vi "3DS Models.vi"(11 "Model":T1=enum."Utah Teapot") -> (3 "Model Out":T2 {"NormalList"."z" format="%.2f"; "NormalList"."y" format="%.2f"; "NormalList"."x" format="%.2f"; "VertexList"."z" format="%.2f"; "VertexList"."y" format="%.2f"; "VertexList"."x" format="%.2f"})   [LabVIEW 2026, in "XRay Part Sample.lvclass"]
uses:
  XRay Part Sample.lvclass
  <vilib>/picture/3D Picture Control/Old 3D Toolkit.llb/model.ctl
  <vilib>/picture/3D Picture Control/Old 3D Toolkit.llb/point3f.ctl
  <vilib>/picture/3D Picture Control/Old 3D Toolkit.llb/VertexMode.ctl
  3D utilities/3DS Models.ctl
  <vilib>/picture/3D Picture Control/NI_Old 3D Toolkit.lvlib
  3D utilities/3D utilities.lvlib
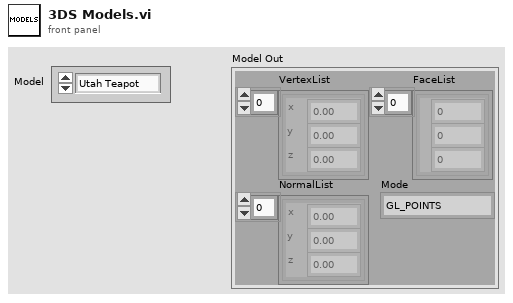
[diagram p1: front panel]
types:
  T1 = typedef "3DS Models.ctl" = enum16{"ASTM E2597 Step Wedge", "NI Bottle", "Utah Teapot", "Utah Teapot (Low Res)", "My Cube", "Tree", "Tree 2", "FreeCAD Sample", "Schenkel", "Bunny", "Corona Virus", "Corona Virus (Low Res)", "Offset"}
  T2 = typedef "NI_3D Picture Control.lvlib/NI_Old 3D Toolkit.lvlib/model.ctl" = cluster{"VertexList":T3[], "FaceList":cluster{"v1":i32, "v2":i32, "v3":i32}[], "NormalList":T3[], "Mode":T4}
  T3 = typedef "NI_3D Picture Control.lvlib/NI_Old 3D Toolkit.lvlib/point3f.ctl" = cluster{"x":sgl, "y":sgl, "z":sgl}
  T4 = typedef "NI_3D Picture Control.lvlib/NI_Old 3D Toolkit.lvlib/VertexMode.ctl" = enum16{"GL_POINTS", "GL_LINES", "GL_LINE_LOOP", "GL_LINE_STRIP", "GL_TRIANGLES", "GL_TRIANGLE_STRIP", "GL_TRIANGLE_FAN", "GL_QUADS", "GL_QUAD_STRIP", "GL_POLYGON"}
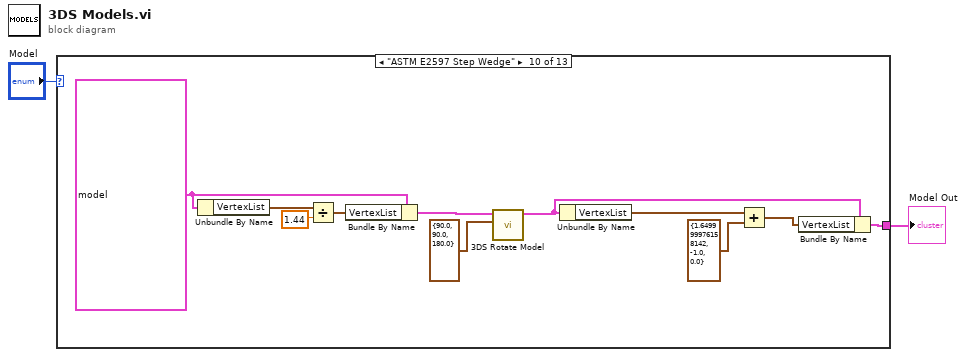
[diagram p0: block diagram]
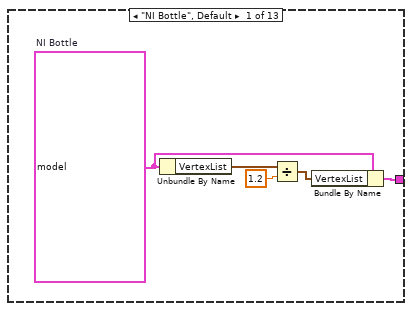
[diagram p2: hidden frame]
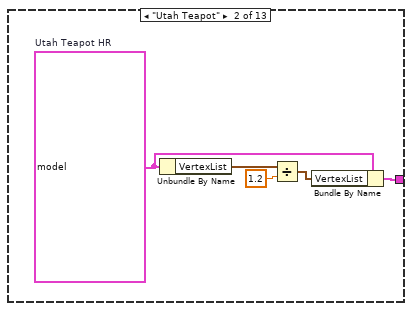
[diagram p3: hidden frame]
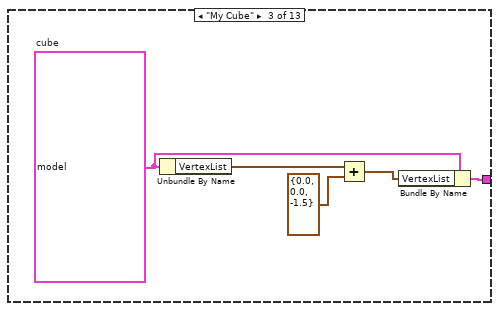
[diagram p4: hidden frame]
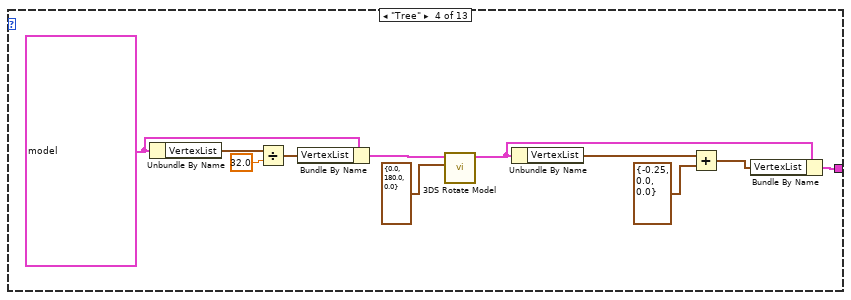
[diagram p5: hidden frame]
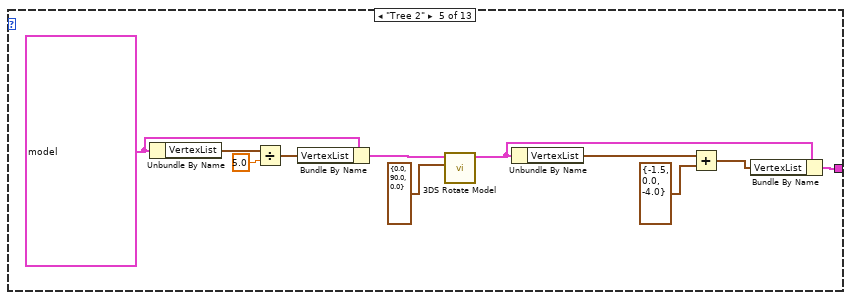
[diagram p6: hidden frame]
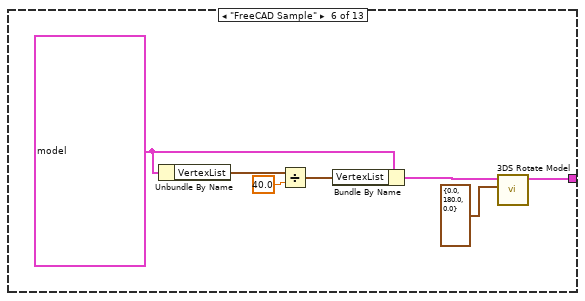
[diagram p7: hidden frame]
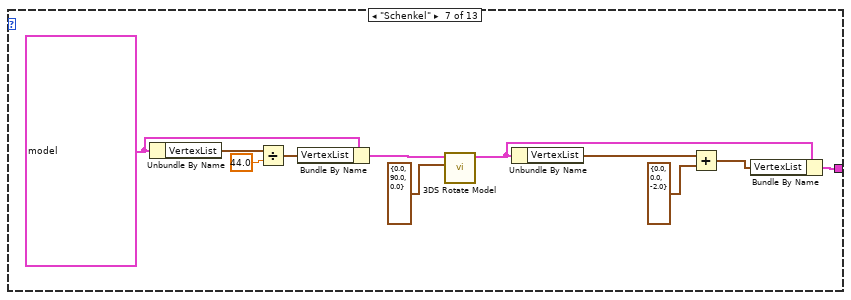
[diagram p8: hidden frame]
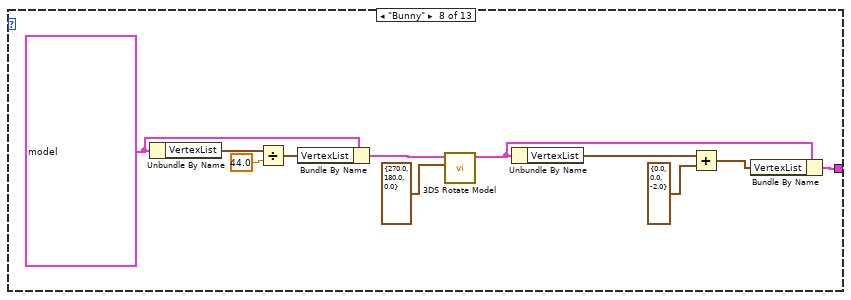
[diagram p9: hidden frame]
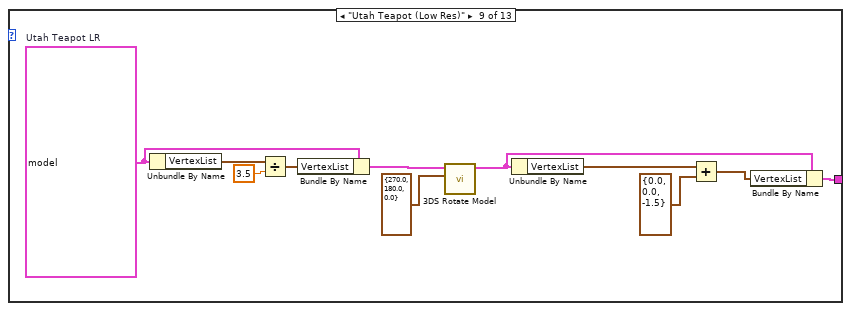
[diagram p10: hidden frame]
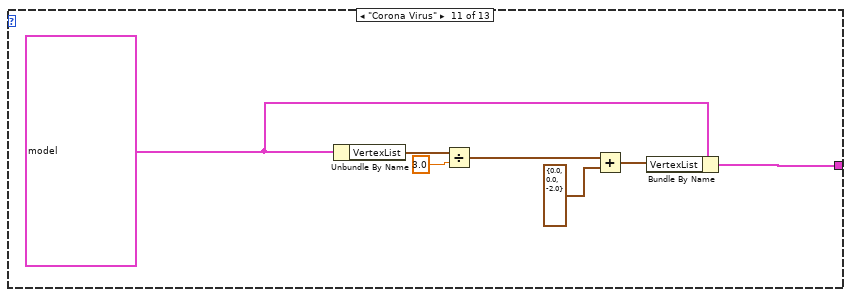
[diagram p11: hidden frame]
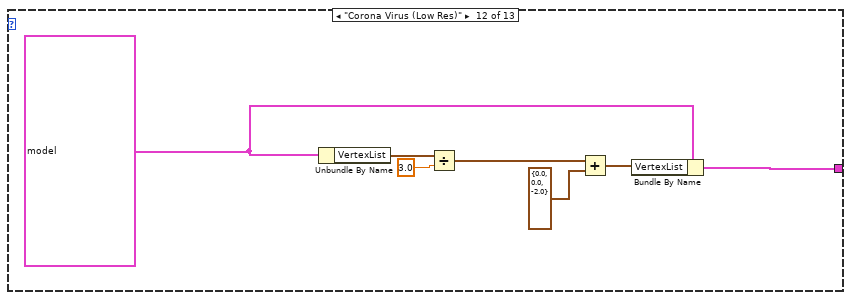
[diagram p12: hidden frame]
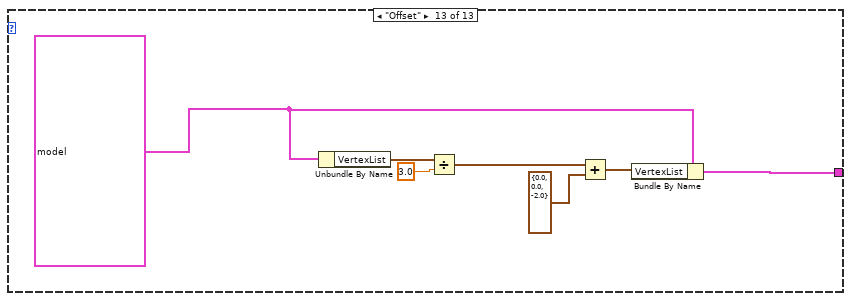
[diagram p13: hidden frame]
diagram:
  n1 = case shown="\"ASTM E2597 Step Wedge\"" "Model" {
    tunnel: [w4 w9 w14 w18 w29 w42 w47 w59 w70 w81 w93 w98 w106] -> w2
    frame "NI Bottle", Default {
      w3 = T2 data[104174B]  # NI Bottle
      n2 = Unbundle By Name(w3) -> ("VertexList"=w7:T3[])
      n3 = Divide(x=w7, y=1.2) -> (x/y=w5:cluster{"x":dbl, "y":dbl, "z":dbl}[])
      n4 = Bundle By Name(cluster=w3, "VertexList"=w5) -> (w4:T2)
    }
    frame "Utah Teapot" {
      w8 = T2 {"VertexList"=array[28314 elements], "FaceList"=array[9438 elements], "NormalList"=array[28314 elements], "Mode"=enum."GL_TRIANGLES"}  # Utah Teapot HR
      n5 = Unbundle By Name(w8) -> ("VertexList"=w12:T3[])
      n6 = Divide(x=w12, y=1.2) -> (x/y=w10:cluster{"x":dbl, "y":dbl, "z":dbl}[])
      n7 = Bundle By Name(cluster=w8, "VertexList"=w10) -> (w9:T2)
    }
    frame "My Cube" {
      w15 = T2 {"VertexList"=[{"x"=1.0, "y"=1.0, "z"=-1.0}, {"x"=1.0, "y"=-1.0, "z"=-1.0}, {"x"=-1.0000001, "y"=-0.9999998, "z"=-1.0}, {"x"=-1.0000001, "y"=-0.9999998, "z"=-1.0}, {"x"=-0.99999964, "y"=1.0000004, "z"=-1.0}, {"x"=1.0, "y"=0.99999994, "z"=-1.0}, {"x"=1.0000005, "y"=0.99999946, "z"=1.0}, {"x"=-0.99999994, "y"=1.0, "z"=1.0}, {"x"=-1.0000004, "y"=-0.99999964, "z"=1.0}, {"x"=-1.0000004, "y"=-0.99999964, "z"=1.0}, {"x"=0.99999934, "y"=-1.0000006, "z"=1.0}, {"x"=1.0000005, "y"=0.99999946, "z"=1.0}, {"x"=1.0, "y"=0.99999994, "z"=-1.0}, {"x"=1.0000005, "y"=0.99999946, "z"=1.0}, {"x"=0.99999934, "y"=-1.0000006, "z"=1.0}, {"x"=0.99999934, "y"=-1.0000006, "z"=1.0}, {"x"=1.0, "y"=-1.0, "z"=-1.0}, {"x"=1.0, "y"=0.99999994, "z"=-1.0}, {"x"=1.0, "y"=-1.0, "z"=-1.0}, {"x"=0.99999934, "y"=-1.0000006, "z"=1.0}, {"x"=-1.0000004, "y"=-0.99999964, "z"=1.0}, {"x"=-1.0000004, "y"=-0.99999964, "z"=1.0}, {"x"=-1.0000001, "y"=-0.9999998, "z"=-1.0}, {"x"=1.0, "y"=-1.0, "z"=-1.0}, {"x"=-1.0000001, "y"=-0.9999998, "z"=-1.0}, {"x"=-1.0000004, "y"=-0.99999964, "z"=1.0}, {"x"=-0.99999994, "y"=1.0, "z"=1.0}, {"x"=-0.99999994, "y"=1.0, "z"=1.0}, {"x"=-0.99999964, "y"=1.0000004, "z"=-1.0}, {"x"=-1.0000001, "y"=-0.9999998, "z"=-1.0}, {"x"=1.0000005, "y"=0.99999946, "z"=1.0}, {"x"=1.0, "y"=0.99999994, "z"=-1.0}, {"x"=-0.99999964, "y"=1.0000004, "z"=-1.0}, {"x"=-0.99999964, "y"=1.0000004, "z"=-1.0}, {"x"=-0.99999994, "y"=1.0, "z"=1.0}, {"x"=1.0000005, "y"=0.99999946, "z"=1.0}], "FaceList"=[{"v1"=0, "v2"=1, "v3"=2}, {"v1"=3, "v2"=4, "v3"=5}, {"v1"=6, "v2"=7, "v3"=8}, {"v1"=9, "v2"=10, "v3"=11}, {"v1"=12, "v2"=13, "v3"=14}, {"v1"=15, "v2"=16, "v3"=17}, {"v1"=18, "v2"=19, "v3"=20}, {"v1"=21, "v2"=22, "v3"=23}, {"v1"=24, "v2"=25, "v3"=26}, {"v1"=27, "v2"=28, "v3"=29}, {"v1"=30, "v2"=31, "v3"=32}, {"v1"=33, "v2"=34, "v3"=35}], "NormalList"=[{"x"=0.0, "y"=0.0, "z"=-1.0}, {"x"=-2.9802326e-08, "y"=0.0, "z"=-1.0}, {"x"=-2.9802326e-08, "y"=0.0, "z"=-1.0}, {"x"=2.9802326e-08, "y"=0.0, "z"=-1.0}, {"x"=2.9802326e-08, "y"=0.0, "z"=-1.0}, {"x"=2.9802326e-08, "y"=0.0, "z"=-1.0}, {"x"=5.9604638e-08, "y"=0.0, "z"=1.0}, {"x"=5.9604638e-08, "y"=0.0, "z"=1.0}, {"x"=5.9604638e-08, "y"=0.0, "z"=1.0}, {"x"=0.0, "y"=0.0, "z"=1.0}, {"x"=1.0, "y"=0.0, "z"=1.0}, {"x"=0.0, "y"=0.0, "z"=1.0}, {"x"=1.0, "y"=-5.9604645e-07, "z"=-2.3841872e-07}, {"x"=1.0, "y"=-5.9604645e-07, "z"=-2.3841872e-07}, {"x"=1.0, "y"=-5.9604645e-07, "z"=-2.3841872e-07}, {"x"=1.0, "y"=0.0, "z"=3.2782552e-07}, {"x"=1.0, "y"=0.0, "z"=3.2782552e-07}, {"x"=1.0, "y"=0.0, "z"=3.2782552e-07}, {"x"=-4.768373e-07, "y"=-1.0, "z"=-3.5762795e-07}, {"x"=-4.768373e-07, "y"=-1.0, "z"=-3.5762795e-07}, {"x"=-4.768373e-07, "y"=-1.0, "z"=-3.5762795e-07}, {"x"=-8.940697e-08, "y"=-1.0, "z"=0.0}, {"x"=-8.940697e-08, "y"=-1.0, "z"=0.0}, {"x"=-8.940697e-08, "y"=-1.0, "z"=0.0}, {"x"=-1.0, "y"=2.3841864e-07, "z"=-1.1920932e-07}, {"x"=-1.0, "y"=2.3841864e-07, "z"=-1.1920932e-07}, {"x"=-1.0, "y"=2.3841864e-07, "z"=-1.1920932e-07}, {"x"=-1.0, "y"=2.3841855e-07, "z"=-1.4901157e-07}, {"x"=-1.0, "y"=2.3841855e-07, "z"=-1.4901157e-07}, {"x"=-1.0, "y"=2.3841855e-07, "z"=-1.4901157e-07}, {"x"=2.0861631e-07, "y"=1.0, "z"=2.9802328e-07}, {"x"=2.0861631e-07, "y"=1.0, "z"=2.9802328e-07}, {"x"=2.0861631e-07, "y"=1.0, "z"=2.9802328e-07}, {"x"=2.6822084e-07, "y"=1.0, "z"=0.0}, {"x"=2.6822084e-07, "y"=1.0, "z"=0.0}, {"x"=2.6822084e-07, "y"=1.0, "z"=0.0}], "Mode"=enum."GL_TRIANGLES"}  # cube
      n8 = Unbundle By Name(w15) -> ("VertexList"=w17:T3[])
      n9 = Add(x=w17, y=T3 {"x"=0.0, "y"=0.0, "z"=-1.5} ("point3f")) -> (x+y=w13:T3[])
      n10 = Bundle By Name(cluster=w15, "VertexList"=w13) -> (w14:T2)
    }
    frame "Tree" {
      w26 = T2 data[30086B] ("Model Out")
      n11 = Unbundle By Name(w26) -> ("VertexList"=w28:T3[])
      n12 = Divide(x=w28, y=32.0) -> (x/y=w25:cluster{"x":dbl, "y":dbl, "z":dbl}[])
      n13 = Bundle By Name(cluster=w26, "VertexList"=w25) -> (w24:T2)
      n14 = call "3DS Rotate Model.vi"("Euler Angles"=cluster{"phi":dbl, "theta":dbl, "psi":dbl} {"phi"=0.0, "theta"=180.0, "psi"=0.0}, "model in"=w24) -> ("model out"=w19:T2)  [unwired: 9 in]
      n15 = Unbundle By Name(w19) -> ("VertexList"=w22:T3[])
      n16 = Add(x=w22, y=T3 {"x"=-0.25, "y"=0.0, "z"=0.0} ("point3f")) -> (x+y=w20:T3[])
      n17 = Bundle By Name(cluster=w19, "VertexList"=w20) -> (w18:T2)
    }
    frame "Tree 2" {
      w34 = T2 {"VertexList"=[{"x"=6.249929, "y"=-20.00003, "z"=0.0}, {"x"=7.766701, "y"=-20.00003, "z"=0.0}, {"x"=6.249929, "y"=-20.00003, "z"=1.0666667}, {"x"=6.249929, "y"=-20.00003, "z"=1.0666667}, {"x"=7.766701, "y"=-20.00003, "z"=0.0}, {"x"=7.766701, "y"=-20.00003, "z"=1.0666667}, {"x"=6.249929, "y"=-18.000015, "z"=0.0}, {"x"=6.249929, "y"=-20.00003, "z"=0.0}, {"x"=6.249929, "y"=-18.000015, "z"=1.0666667}, {"x"=6.249929, "y"=-18.000015, "z"=1.0666667}, {"x"=6.249929, "y"=-20.00003, "z"=0.0}, {"x"=6.249929, "y"=-20.00003, "z"=1.0666667}, {"x"=0.0, "y"=-18.000015, "z"=0.0}, {"x"=6.249929, "y"=-18.000015, "z"=0.0}, {"x"=0.0, "y"=-18.000015, "z"=1.0666667}, {"x"=0.0, "y"=-18.000015, "z"=1.0666667}, {"x"=6.249929, "y"=-18.000015, "z"=0.0}, {"x"=6.249929, "y"=-18.000015, "z"=1.0666667}, {"x"=4.166658, "y"=-12.000089, "z"=0.0}, {"x"=0.0, "y"=-18.000015, "z"=0.0}, {"x"=4.166658, "y"=-12.000089, "z"=1.0666667}, {"x"=4.166658, "y"=-12.000089, "z"=1.0666667}, {"x"=0.0, "y"=-18.000015, "z"=0.0}, {"x"=0.0, "y"=-18.000015, "z"=1.0666667}, {"x"=2.0832703, "y"=-12.000089, "z"=0.0}, {"x"=4.166658, "y"=-12.000089, "z"=0.0}, {"x"=2.0832703, "y"=-12.000089, "z"=1.0666667}, {"x"=2.0832703, "y"=-12.000089, "z"=1.0666667}, {"x"=4.166658, "y"=-12.000089, "z"=0.0}, {"x"=4.166658, "y"=-12.000089, "z"=1.0666667}, {"x"=6.249929, "y"=-6.0000443, "z"=0.0}, {"x"=2.0832703, "y"=-12.000089, "z"=0.0}, {"x"=6.249929, "y"=-6.0000443, "z"=1.0666667}, {"x"=6.249929, "y"=-6.0000443, "z"=1.0666667}, {"x"=2.0832703, "y"=-12.000089, "z"=0.0}, {"x"=2.0832703, "y"=-12.000089, "z"=1.0666667}, {"x"=4.166658, "y"=-6.0000443, "z"=0.0}, {"x"=6.249929, "y"=-6.0000443, "z"=0.0}, {"x"=4.166658, "y"=-6.0000443, "z"=1.0666667}, {"x"=4.166658, "y"=-6.0000443, "z"=1.0666667}, {"x"=6.249929, "y"=-6.0000443, "z"=0.0}, {"x"=6.249929, "y"=-6.0000443, "z"=1.0666667}, {"x"=8.333434, "y"=-6.1724626e-07, "z"=0.0}, {"x"=4.166658, "y"=-6.0000443, "z"=0.0}, {"x"=8.333434, "y"=-6.1724626e-07, "z"=1.0666667}, {"x"=8.333434, "y"=-6.1724626e-07, "z"=1.0666667}, {"x"=4.166658, "y"=-6.0000443, "z"=0.0}, {"x"=4.166658, "y"=-6.0000443, "z"=1.0666667}, {"x"=12.499976, "y"=-6.0000443, "z"=0.0}, {"x"=8.333434, "y"=-6.1724626e-07, "z"=0.0}, {"x"=12.499976, "y"=-6.0000443, "z"=1.0666667}, {"x"=12.499976, "y"=-6.0000443, "z"=1.0666667}, {"x"=8.333434, "y"=-6.1724626e-07, "z"=0.0}, {"x"=8.333434, "y"=-6.1724626e-07, "z"=1.0666667}, {"x"=10.416705, "y"=-6.0000443, "z"=0.0}, {"x"=12.499976, "y"=-6.0000443, "z"=0.0}, {"x"=10.416705, "y"=-6.0000443, "z"=1.0666667}, {"x"=10.416705, "y"=-6.0000443, "z"=1.0666667}, {"x"=12.499976, "y"=-6.0000443, "z"=0.0}, {"x"=12.499976, "y"=-6.0000443, "z"=1.0666667}, {"x"=14.583245, "y"=-12.000089, "z"=0.0}, {"x"=10.416705, "y"=-6.0000443, "z"=0.0}, {"x"=14.583245, "y"=-12.000089, "z"=1.0666667}, {"x"=14.583245, "y"=-12.000089, "z"=1.0666667}, {"x"=10.416705, "y"=-6.0000443, "z"=0.0}, {"x"=10.416705, "y"=-6.0000443, "z"=1.0666667}, {"x"=12.499976, "y"=-12.000089, "z"=0.0}, {"x"=14.583245, "y"=-12.000089, "z"=0.0}, {"x"=12.499976, "y"=-12.000089, "z"=1.0666667}, {"x"=12.499976, "y"=-12.000089, "z"=1.0666667}, {"x"=14.583245, "y"=-12.000089, "z"=0.0}, {"x"=14.583245, "y"=-12.000089, "z"=1.0666667}, {"x"=16.66675, "y"=-18.000015, "z"=0.0}, {"x"=12.499976, "y"=-12.000089, "z"=0.0}, {"x"=16.66675, "y"=-18.000015, "z"=1.0666667}, {"x"=16.66675, "y"=-18.000015, "z"=1.0666667}, {"x"=12.499976, "y"=-12.000089, "z"=0.0}, {"x"=12.499976, "y"=-12.000089, "z"=1.0666667}, {"x"=10.416705, "y"=-18.000015, "z"=0.0}, {"x"=16.66675, "y"=-18.000015, "z"=0.0}, {"x"=10.416705, "y"=-18.000015, "z"=1.0666667}, {"x"=10.416705, "y"=-18.000015, "z"=1.0666667}, {"x"=16.66675, "y"=-18.000015, "z"=0.0}, {"x"=16.66675, "y"=-18.000015, "z"=1.0666667}, {"x"=10.416705, "y"=-20.00003, "z"=0.0}, {"x"=10.416705, "y"=-18.000015, "z"=0.0}, {"x"=10.416705, "y"=-20.00003, "z"=1.0666667}, {"x"=10.416705, "y"=-20.00003, "z"=1.0666667}, {"x"=10.416705, "y"=-18.000015, "z"=0.0}, {"x"=10.416705, "y"=-18.000015, "z"=1.0666667}, {"x"=8.90005, "y"=-20.00003, "z"=0.0}, {"x"=10.416705, "y"=-20.00003, "z"=0.0}, {"x"=8.90005, "y"=-20.00003, "z"=1.0666667}, {"x"=8.90005, "y"=-20.00003, "z"=1.0666667}, {"x"=10.416705, "y"=-20.00003, "z"=0.0}, {"x"=10.416705, "y"=-20.00003, "z"=1.0666667}, {"x"=8.90005, "y"=-9.966741, "z"=0.0}, {"x"=8.90005, "y"=-20.00003, "z"=0.0}, {"x"=8.90005, "y"=-9.966741, "z"=1.0666667}, {"x"=8.90005, "y"=-9.966741, "z"=1.0666667}, {"x"=8.90005, "y"=-20.00003, "z"=0.0}, {"x"=8.90005, "y"=-20.00003, "z"=1.0666667}, {"x"=7.766701, "y"=-9.966741, "z"=0.0}, {"x"=8.90005, "y"=-9.966741, "z"=0.0}, {"x"=7.766701, "y"=-9.966741, "z"=1.0666667}, {"x"=7.766701, "y"=-9.966741, "z"=1.0666667}, {"x"=8.90005, "y"=-9.966741, "z"=0.0}, {"x"=8.90005, "y"=-9.966741, "z"=1.0666667}, {"x"=7.766701, "y"=-20.00003, "z"=0.0}, {"x"=7.766701, "y"=-9.966741, "z"=0.0}, {"x"=7.766701, "y"=-20.00003, "z"=1.0666667}, {"x"=7.766701, "y"=-20.00003, "z"=1.0666667}, {"x"=7.766701, "y"=-9.966741, "z"=0.0}, {"x"=7.766701, "y"=-9.966741, "z"=1.0666667}, {"x"=6.249929, "y"=-20.00003, "z"=1.0666667}, {"x"=7.766701, "y"=-20.00003, "z"=1.0666667}, {"x"=6.249929, "y"=-18.000015, "z"=1.0666667}, {"x"=6.249929, "y"=-18.000015, "z"=1.0666667}, {"x"=7.766701, "y"=-20.00003, "z"=1.0666667}, {"x"=7.766701, "y"=-9.966741, "z"=1.0666667}, {"x"=6.249929, "y"=-18.000015, "z"=1.0666667}, {"x"=7.766701, "y"=-9.966741, "z"=1.0666667}, {"x"=4.166658, "y"=-12.000089, "z"=1.0666667}, {"x"=4.166658, "y"=-12.000089, "z"=1.0666667}, {"x"=7.766701, "y"=-9.966741, "z"=1.0666667}, {"x"=6.249929, "y"=-6.0000443, "z"=1.0666667}, {"x"=4.166658, "y"=-12.000089, "z"=1.0666667}, {"x"=6.249929, "y"=-6.0000443, "z"=1.0666667}, {"x"=2.0832703, "y"=-12.000089, "z"=1.0666667}, {"x"=6.249929, "y"=-6.0000443, "z"=1.0666667}, {"x"=7.766701, "y"=-9.966741, "z"=1.0666667}, {"x"=10.416705, "y"=-6.0000443, "z"=1.0666667}, {"x"=10.416705, "y"=-6.0000443, "z"=1.0666667}, {"x"=7.766701, "y"=-9.966741, "z"=1.0666667}, {"x"=8.90005, "y"=-9.966741, "z"=1.0666667}, {"x"=10.416705, "y"=-6.0000443, "z"=1.0666667}, {"x"=8.90005, "y"=-9.966741, "z"=1.0666667}, {"x"=12.499976, "y"=-12.000089, "z"=1.0666667}, {"x"=12.499976, "y"=-12.000089, "z"=1.0666667}, {"x"=8.90005, "y"=-9.966741, "z"=1.0666667}, {"x"=10.416705, "y"=-18.000015, "z"=1.0666667}, {"x"=12.499976, "y"=-12.000089, "z"=1.0666667}, {"x"=10.416705, "y"=-18.000015, "z"=1.0666667}, {"x"=16.66675, "y"=-18.000015, "z"=1.0666667}, {"x"=8.90005, "y"=-9.966741, "z"=1.0666667}, {"x"=8.90005, "y"=-20.00003, "z"=1.0666667}, {"x"=10.416705, "y"=-18.000015, "z"=1.0666667}, {"x"=10.416705, "y"=-18.000015, "z"=1.0666667}, {"x"=8.90005, "y"=-20.00003, "z"=1.0666667}, {"x"=10.416705, "y"=-20.00003, "z"=1.0666667}, {"x"=12.499976, "y"=-12.000089, "z"=1.0666667}, {"x"=14.583245, "y"=-12.000089, "z"=1.0666667}, {"x"=10.416705, "y"=-6.0000443, "z"=1.0666667}, {"x"=12.499976, "y"=-6.0000443, "z"=1.0666667}, {"x"=8.333434, "y"=-6.1724626e-07, "z"=1.0666667}, {"x"=10.416705, "y"=-6.0000443, "z"=1.0666667}, {"x"=10.416705, "y"=-6.0000443, "z"=1.0666667}, {"x"=8.333434, "y"=-6.1724626e-07, "z"=1.0666667}, {"x"=6.249929, "y"=-6.0000443, "z"=1.0666667}, {"x"=8.333434, "y"=-6.1724626e-07, "z"=1.0666667}, {"x"=4.166658, "y"=-6.0000443, "z"=1.0666667}, {"x"=6.249929, "y"=-6.0000443, "z"=1.0666667}, {"x"=4.166658, "y"=-12.000089, "z"=1.0666667}, {"x"=0.0, "y"=-18.000015, "z"=1.0666667}, {"x"=6.249929, "y"=-18.000015, "z"=1.0666667}, {"x"=7.766701, "y"=-20.00003, "z"=0.0}, {"x"=6.249929, "y"=-18.000015, "z"=0.0}, {"x"=7.766701, "y"=-9.966741, "z"=0.0}, {"x"=7.766701, "y"=-9.966741, "z"=0.0}, {"x"=6.249929, "y"=-18.000015, "z"=0.0}, {"x"=4.166658, "y"=-12.000089, "z"=0.0}, {"x"=7.766701, "y"=-9.966741, "z"=0.0}, {"x"=4.166658, "y"=-12.000089, "z"=0.0}, {"x"=6.249929, "y"=-6.0000443, "z"=0.0}, {"x"=6.249929, "y"=-6.0000443, "z"=0.0}, {"x"=4.166658, "y"=-12.000089, "z"=0.0}, {"x"=2.0832703, "y"=-12.000089, "z"=0.0}, {"x"=7.766701, "y"=-20.00003, "z"=0.0}, {"x"=6.249929, "y"=-20.00003, "z"=0.0}, {"x"=6.249929, "y"=-18.000015, "z"=0.0}, {"x"=6.249929, "y"=-18.000015, "z"=0.0}, {"x"=0.0, "y"=-18.000015, "z"=0.0}, {"x"=4.166658, "y"=-12.000089, "z"=0.0}, {"x"=4.166658, "y"=-6.0000443, "z"=0.0}, {"x"=8.333434, "y"=-6.1724626e-07, "z"=0.0}, {"x"=6.249929, "y"=-6.0000443, "z"=0.0}, {"x"=6.249929, "y"=-6.0000443, "z"=0.0}, {"x"=8.333434, "y"=-6.1724626e-07, "z"=0.0}, {"x"=10.416705, "y"=-6.0000443, "z"=0.0}, {"x"=6.249929, "y"=-6.0000443, "z"=0.0}, {"x"=10.416705, "y"=-6.0000443, "z"=0.0}, {"x"=7.766701, "y"=-9.966741, "z"=0.0}, {"x"=7.766701, "y"=-9.966741, "z"=0.0}, {"x"=10.416705, "y"=-6.0000443, "z"=0.0}, {"x"=8.90005, "y"=-9.966741, "z"=0.0}, {"x"=8.90005, "y"=-9.966741, "z"=0.0}, {"x"=10.416705, "y"=-6.0000443, "z"=0.0}, {"x"=12.499976, "y"=-12.000089, "z"=0.0}, {"x"=8.90005, "y"=-9.966741, "z"=0.0}, {"x"=12.499976, "y"=-12.000089, "z"=0.0}, {"x"=10.416705, "y"=-18.000015, "z"=0.0}, {"x"=10.416705, "y"=-18.000015, "z"=0.0}, {"x"=12.499976, "y"=-12.000089, "z"=0.0}, {"x"=16.66675, "y"=-18.000015, "z"=0.0}, {"x"=8.333434, "y"=-6.1724626e-07, "z"=0.0}, {"x"=12.499976, "y"=-6.0000443, "z"=0.0}, {"x"=10.416705, "y"=-6.0000443, "z"=0.0}, {"x"=10.416705, "y"=-6.0000443, "z"=0.0}, {"x"=14.583245, "y"=-12.000089, "z"=0.0}, {"x"=12.499976, "y"=-12.000089, "z"=0.0}, {"x"=10.416705, "y"=-20.00003, "z"=0.0}, {"x"=8.90005, "y"=-20.00003, "z"=0.0}, {"x"=10.416705, "y"=-18.000015, "z"=0.0}, {"x"=10.416705, "y"=-18.000015, "z"=0.0}, {"x"=8.90005, "y"=-20.00003, "z"=0.0}, {"x"=8.90005, "y"=-9.966741, "z"=0.0}], "FaceList"=[{"v1"=0, "v2"=1, "v3"=2}, {"v1"=3, "v2"=4, "v3"=5}, {"v1"=6, "v2"=7, "v3"=8}, {"v1"=9, "v2"=10, "v3"=11}, {"v1"=12, "v2"=13, "v3"=14}, {"v1"=15, "v2"=16, "v3"=17}, {"v1"=18, "v2"=19, "v3"=20}, {"v1"=21, "v2"=22, "v3"=23}, {"v1"=24, "v2"=25, "v3"=26}, {"v1"=27, "v2"=28, "v3"=29}, {"v1"=30, "v2"=31, "v3"=32}, {"v1"=33, "v2"=34, "v3"=35}, {"v1"=36, "v2"=37, "v3"=38}, {"v1"=39, "v2"=40, "v3"=41}, {"v1"=42, "v2"=43, "v3"=44}, {"v1"=45, "v2"=46, "v3"=47}, {"v1"=48, "v2"=49, "v3"=50}, {"v1"=51, "v2"=52, "v3"=53}, {"v1"=54, "v2"=55, "v3"=56}, {"v1"=57, "v2"=58, "v3"=59}, {"v1"=60, "v2"=61, "v3"=62}, {"v1"=63, "v2"=64, "v3"=65}, {"v1"=66, "v2"=67, "v3"=68}, {"v1"=69, "v2"=70, "v3"=71}, {"v1"=72, "v2"=73, "v3"=74}, {"v1"=75, "v2"=76, "v3"=77}, {"v1"=78, "v2"=79, "v3"=80}, {"v1"=81, "v2"=82, "v3"=83}, {"v1"=84, "v2"=85, "v3"=86}, {"v1"=87, "v2"=88, "v3"=89}, {"v1"=90, "v2"=91, "v3"=92}, {"v1"=93, "v2"=94, "v3"=95}, {"v1"=96, "v2"=97, "v3"=98}, {"v1"=99, "v2"=100, "v3"=101}, {"v1"=102, "v2"=103, "v3"=104}, {"v1"=105, "v2"=106, "v3"=107}, {"v1"=108, "v2"=109, "v3"=110}, {"v1"=111, "v2"=112, "v3"=113}, {"v1"=114, "v2"=115, "v3"=116}, {"v1"=117, "v2"=118, "v3"=119}, {"v1"=120, "v2"=121, "v3"=122}, {"v1"=123, "v2"=124, "v3"=125}, {"v1"=126, "v2"=127, "v3"=128}, {"v1"=129, "v2"=130, "v3"=131}, {"v1"=132, "v2"=133, "v3"=134}, {"v1"=135, "v2"=136, "v3"=137}, {"v1"=138, "v2"=139, "v3"=140}, {"v1"=141, "v2"=142, "v3"=143}, {"v1"=144, "v2"=145, "v3"=146}, {"v1"=147, "v2"=148, "v3"=149}, {"v1"=150, "v2"=151, "v3"=152}, {"v1"=153, "v2"=154, "v3"=155}, {"v1"=156, "v2"=157, "v3"=158}, {"v1"=159, "v2"=160, "v3"=161}, {"v1"=162, "v2"=163, "v3"=164}, {"v1"=165, "v2"=166, "v3"=167}, {"v1"=168, "v2"=169, "v3"=170}, {"v1"=171, "v2"=172, "v3"=173}, {"v1"=174, "v2"=175, "v3"=176}, {"v1"=177, "v2"=178, "v3"=179}, {"v1"=180, "v2"=181, "v3"=182}, {"v1"=183, "v2"=184, "v3"=185}, {"v1"=186, "v2"=187, "v3"=188}, {"v1"=189, "v2"=190, "v3"=191}, {"v1"=192, "v2"=193, "v3"=194}, {"v1"=195, "v2"=196, "v3"=197}, {"v1"=198, "v2"=199, "v3"=200}, {"v1"=201, "v2"=202, "v3"=203}, {"v1"=204, "v2"=205, "v3"=206}, {"v1"=207, "v2"=208, "v3"=209}, {"v1"=210, "v2"=211, "v3"=212}, {"v1"=213, "v2"=214, "v3"=215}], "NormalList"=[{"x"=-1.5615233e-15, "y"=-1.0, "z"=0.0}, {"x"=-1.5615233e-15, "y"=-1.0, "z"=0.0}, {"x"=-1.5615233e-15, "y"=-1.0, "z"=0.0}, {"x"=-1.5615233e-15, "y"=-1.0, "z"=0.0}, {"x"=-1.5615233e-15, "y"=-1.0, "z"=0.0}, {"x"=-1.5615233e-15, "y"=-1.0, "z"=0.0}, {"x"=-1.0, "y"=0.0, "z"=0.0}, {"x"=-1.0, "y"=0.0, "z"=0.0}, {"x"=-1.0, "y"=0.0, "z"=0.0}, {"x"=-1.0, "y"=-0.0, "z"=0.0}, {"x"=-1.0, "y"=-0.0, "z"=0.0}, {"x"=-1.0, "y"=-0.0, "z"=0.0}, {"x"=0.0, "y"=-1.0, "z"=0.0}, {"x"=0.0, "y"=-1.0, "z"=0.0}, {"x"=0.0, "y"=-1.0, "z"=0.0}, {"x"=0.0, "y"=-1.0, "z"=0.0}, {"x"=0.0, "y"=-1.0, "z"=0.0}, {"x"=0.0, "y"=-1.0, "z"=0.0}, {"x"=-0.82136726, "y"=0.5703997, "z"=0.0}, {"x"=-0.82136726, "y"=0.5703997, "z"=0.0}, {"x"=-0.82136726, "y"=0.5703997, "z"=0.0}, {"x"=-0.82136726, "y"=0.5703997, "z"=0.0}, {"x"=-0.82136726, "y"=0.5703997, "z"=0.0}, {"x"=-0.82136726, "y"=0.5703997, "z"=0.0}, {"x"=0.0, "y"=-1.0, "z"=0.0}, {"x"=0.0, "y"=-1.0, "z"=0.0}, {"x"=0.0, "y"=-1.0, "z"=0.0}, {"x"=0.0, "y"=-1.0, "z"=0.0}, {"x"=0.0, "y"=-1.0, "z"=0.0}, {"x"=0.0, "y"=-1.0, "z"=0.0}, {"x"=-0.8213725, "y"=0.57039213, "z"=0.0}, {"x"=-0.8213725, "y"=0.57039213, "z"=0.0}, {"x"=-0.8213725, "y"=0.57039213, "z"=0.0}, {"x"=-0.8213725, "y"=0.57039213, "z"=0.0}, {"x"=-0.8213725, "y"=0.57039213, "z"=0.0}, {"x"=-0.8213725, "y"=0.57039213, "z"=0.0}, {"x"=0.0, "y"=-1.0, "z"=0.0}, {"x"=0.0, "y"=-1.0, "z"=0.0}, {"x"=0.0, "y"=-1.0, "z"=0.0}, {"x"=0.0, "y"=-1.0, "z"=0.0}, {"x"=0.0, "y"=-1.0, "z"=0.0}, {"x"=0.0, "y"=-1.0, "z"=0.0}, {"x"=-0.82136494, "y"=0.5704031, "z"=3.9579663e-16}, {"x"=-0.82136494, "y"=0.5704031, "z"=3.9579663e-16}, {"x"=-0.82136494, "y"=0.5704031, "z"=3.9579663e-16}, {"x"=-0.82136494, "y"=0.5704031, "z"=0.0}, {"x"=-0.82136494, "y"=0.5704031, "z"=0.0}, {"x"=-0.82136494, "y"=0.5704031, "z"=0.0}, {"x"=0.82137996, "y"=0.57038146, "z"=-0.0}, {"x"=0.82137996, "y"=0.57038146, "z"=-0.0}, {"x"=0.82137996, "y"=0.57038146, "z"=-0.0}, {"x"=0.82137996, "y"=0.57038146, "z"=8.105851e-16}, {"x"=0.82137996, "y"=0.57038146, "z"=8.105851e-16}, {"x"=0.82137996, "y"=0.57038146, "z"=8.105851e-16}, {"x"=0.0, "y"=-1.0, "z"=0.0}, {"x"=0.0, "y"=-1.0, "z"=0.0}, {"x"=0.0, "y"=-1.0, "z"=0.0}, {"x"=0.0, "y"=-1.0, "z"=0.0}, {"x"=0.0, "y"=-1.0, "z"=0.0}, {"x"=0.0, "y"=-1.0, "z"=0.0}, {"x"=0.82138, "y"=0.5703813, "z"=-0.0}, {"x"=0.82138, "y"=0.5703813, "z"=-0.0}, {"x"=0.82138, "y"=0.5703813, "z"=-0.0}, {"x"=0.82138, "y"=0.5703813, "z"=0.0}, {"x"=0.82138, "y"=0.5703813, "z"=0.0}, {"x"=0.82138, "y"=0.5703813, "z"=0.0}, {"x"=0.0, "y"=-1.0, "z"=0.0}, {"x"=0.0, "y"=-1.0, "z"=0.0}, {"x"=0.0, "y"=-1.0, "z"=0.0}, {"x"=0.0, "y"=-1.0, "z"=0.0}, {"x"=0.0, "y"=-1.0, "z"=0.0}, {"x"=0.0, "y"=-1.0, "z"=0.0}, {"x"=0.8213597, "y"=0.5704106, "z"=-0.0}, {"x"=0.8213597, "y"=0.5704106, "z"=-0.0}, {"x"=0.8213597, "y"=0.5704106, "z"=-0.0}, {"x"=0.8213597, "y"=0.5704106, "z"=0.0}, {"x"=0.8213597, "y"=0.5704106, "z"=0.0}, {"x"=0.8213597, "y"=0.5704106, "z"=0.0}, {"x"=0.0, "y"=-1.0, "z"=0.0}, {"x"=0.0, "y"=-1.0, "z"=0.0}, {"x"=0.0, "y"=-1.0, "z"=0.0}, {"x"=0.0, "y"=-1.0, "z"=0.0}, {"x"=0.0, "y"=-1.0, "z"=0.0}, {"x"=0.0, "y"=-1.0, "z"=0.0}, {"x"=1.0, "y"=0.0, "z"=0.0}, {"x"=1.0, "y"=0.0, "z"=0.0}, {"x"=1.0, "y"=0.0, "z"=0.0}, {"x"=1.0, "y"=-0.0, "z"=0.0}, {"x"=1.0, "y"=-0.0, "z"=0.0}, {"x"=1.0, "y"=-0.0, "z"=0.0}, {"x"=0.0, "y"=-1.0, "z"=0.0}, {"x"=0.0, "y"=-1.0, "z"=0.0}, {"x"=0.0, "y"=-1.0, "z"=0.0}, {"x"=0.0, "y"=-1.0, "z"=0.0}, {"x"=0.0, "y"=-1.0, "z"=0.0}, {"x"=0.0, "y"=-1.0, "z"=0.0}, {"x"=-1.0, "y"=0.0, "z"=0.0}, {"x"=-1.0, "y"=0.0, "z"=0.0}, {"x"=-1.0, "y"=0.0, "z"=0.0}, {"x"=-1.0, "y"=-0.0, "z"=0.0}, {"x"=-1.0, "y"=-0.0, "z"=0.0}, {"x"=-1.0, "y"=-0.0, "z"=0.0}, {"x"=1.0449013e-15, "y"=-1.0, "z"=0.0}, {"x"=1.0449013e-15, "y"=-1.0, "z"=0.0}, {"x"=1.0449013e-15, "y"=-1.0, "z"=0.0}, {"x"=1.0449013e-15, "y"=-1.0, "z"=0.0}, {"x"=1.0449013e-15, "y"=-1.0, "z"=0.0}, {"x"=1.0449013e-15, "y"=-1.0, "z"=0.0}, {"x"=1.0, "y"=0.0, "z"=0.0}, {"x"=1.0, "y"=0.0, "z"=0.0}, {"x"=1.0, "y"=0.0, "z"=0.0}, {"x"=1.0, "y"=-0.0, "z"=0.0}, {"x"=1.0, "y"=-0.0, "z"=0.0}, {"x"=1.0, "y"=-0.0, "z"=0.0}, {"x"=-0.0, "y"=0.0, "z"=1.0}, {"x"=-0.0, "y"=0.0, "z"=1.0}, {"x"=-0.0, "y"=0.0, "z"=1.0}, {"x"=-0.0, "y"=0.0, "z"=1.0}, {"x"=-0.0, "y"=0.0, "z"=1.0}, {"x"=-0.0, "y"=0.0, "z"=1.0}, {"x"=0.0, "y"=-0.0, "z"=1.0}, {"x"=0.0, "y"=-0.0, "z"=1.0}, {"x"=0.0, "y"=-0.0, "z"=1.0}, {"x"=0.0, "y"=0.0, "z"=1.0}, {"x"=0.0, "y"=0.0, "z"=1.0}, {"x"=0.0, "y"=0.0, "z"=1.0}, {"x"=0.0, "y"=-0.0, "z"=1.0}, {"x"=0.0, "y"=-0.0, "z"=1.0}, {"x"=0.0, "y"=-0.0, "z"=1.0}, {"x"=-0.0, "y"=0.0, "z"=1.0}, {"x"=-0.0, "y"=0.0, "z"=1.0}, {"x"=-0.0, "y"=0.0, "z"=1.0}, {"x"=0.0, "y"=0.0, "z"=1.0}, {"x"=0.0, "y"=0.0, "z"=1.0}, {"x"=0.0, "y"=0.0, "z"=1.0}, {"x"=0.0, "y"=0.0, "z"=1.0}, {"x"=0.0, "y"=0.0, "z"=1.0}, {"x"=0.0, "y"=0.0, "z"=1.0}, {"x"=0.0, "y"=0.0, "z"=1.0}, {"x"=0.0, "y"=0.0, "z"=1.0}, {"x"=0.0, "y"=0.0, "z"=1.0}, {"x"=0.0, "y"=0.0, "z"=1.0}, {"x"=0.0, "y"=0.0, "z"=1.0}, {"x"=0.0, "y"=0.0, "z"=1.0}, {"x"=0.0, "y"=0.0, "z"=1.0}, {"x"=0.0, "y"=0.0, "z"=1.0}, {"x"=0.0, "y"=0.0, "z"=1.0}, {"x"=0.0, "y"=0.0, "z"=1.0}, {"x"=0.0, "y"=0.0, "z"=1.0}, {"x"=0.0, "y"=0.0, "z"=1.0}, {"x"=0.0, "y"=-0.0, "z"=1.0}, {"x"=0.0, "y"=-0.0, "z"=1.0}, {"x"=0.0, "y"=-0.0, "z"=1.0}, {"x"=0.0, "y"=0.0, "z"=1.0}, {"x"=0.0, "y"=0.0, "z"=1.0}, {"x"=0.0, "y"=0.0, "z"=1.0}, {"x"=0.0, "y"=0.0, "z"=1.0}, {"x"=0.0, "y"=0.0, "z"=1.0}, {"x"=0.0, "y"=0.0, "z"=1.0}, {"x"=0.0, "y"=0.0, "z"=1.0}, {"x"=0.0, "y"=0.0, "z"=1.0}, {"x"=0.0, "y"=0.0, "z"=1.0}, {"x"=0.0, "y"=0.0, "z"=1.0}, {"x"=0.0, "y"=0.0, "z"=1.0}, {"x"=0.0, "y"=0.0, "z"=1.0}, {"x"=0.0, "y"=0.0, "z"=-1.0}, {"x"=0.0, "y"=0.0, "z"=-1.0}, {"x"=0.0, "y"=0.0, "z"=-1.0}, {"x"=0.0, "y"=0.0, "z"=-1.0}, {"x"=0.0, "y"=0.0, "z"=-1.0}, {"x"=0.0, "y"=0.0, "z"=-1.0}, {"x"=-0.0, "y"=0.0, "z"=-1.0}, {"x"=-0.0, "y"=0.0, "z"=-1.0}, {"x"=-0.0, "y"=0.0, "z"=-1.0}, {"x"=0.0, "y"=0.0, "z"=-1.0}, {"x"=0.0, "y"=0.0, "z"=-1.0}, {"x"=0.0, "y"=0.0, "z"=-1.0}, {"x"=0.0, "y"=0.0, "z"=-1.0}, {"x"=0.0, "y"=0.0, "z"=-1.0}, {"x"=0.0, "y"=0.0, "z"=-1.0}, {"x"=0.0, "y"=0.0, "z"=-1.0}, {"x"=0.0, "y"=0.0, "z"=-1.0}, {"x"=0.0, "y"=0.0, "z"=-1.0}, {"x"=0.0, "y"=0.0, "z"=-1.0}, {"x"=0.0, "y"=0.0, "z"=-1.0}, {"x"=0.0, "y"=0.0, "z"=-1.0}, {"x"=0.0, "y"=0.0, "z"=-1.0}, {"x"=0.0, "y"=0.0, "z"=-1.0}, {"x"=0.0, "y"=0.0, "z"=-1.0}, {"x"=0.0, "y"=0.0, "z"=-1.0}, {"x"=0.0, "y"=0.0, "z"=-1.0}, {"x"=0.0, "y"=0.0, "z"=-1.0}, {"x"=0.0, "y"=0.0, "z"=-1.0}, {"x"=0.0, "y"=0.0, "z"=-1.0}, {"x"=0.0, "y"=0.0, "z"=-1.0}, {"x"=0.0, "y"=0.0, "z"=-1.0}, {"x"=0.0, "y"=0.0, "z"=-1.0}, {"x"=0.0, "y"=0.0, "z"=-1.0}, {"x"=0.0, "y"=0.0, "z"=-1.0}, {"x"=0.0, "y"=0.0, "z"=-1.0}, {"x"=0.0, "y"=0.0, "z"=-1.0}, {"x"=0.0, "y"=0.0, "z"=-1.0}, {"x"=0.0, "y"=0.0, "z"=-1.0}, {"x"=0.0, "y"=0.0, "z"=-1.0}, {"x"=0.0, "y"=0.0, "z"=-1.0}, {"x"=0.0, "y"=0.0, "z"=-1.0}, {"x"=0.0, "y"=0.0, "z"=-1.0}, {"x"=0.0, "y"=0.0, "z"=-1.0}, {"x"=0.0, "y"=0.0, "z"=-1.0}, {"x"=0.0, "y"=0.0, "z"=-1.0}, {"x"=0.0, "y"=0.0, "z"=-1.0}, {"x"=0.0, "y"=0.0, "z"=-1.0}, {"x"=0.0, "y"=0.0, "z"=-1.0}, {"x"=-0.0, "y"=0.0, "z"=-1.0}, {"x"=-0.0, "y"=0.0, "z"=-1.0}, {"x"=-0.0, "y"=0.0, "z"=-1.0}], "Mode"=enum."GL_TRIANGLES"} ("Object Out")
      n18 = Unbundle By Name(w34) -> ("VertexList"=w39:T3[])
      n19 = Divide(x=w39, y=5.0) -> (x/y=w37:cluster{"x":dbl, "y":dbl, "z":dbl}[])
      n20 = Bundle By Name(cluster=w34, "VertexList"=w37) -> (w36:T2)
      n21 = call "3DS Rotate Model.vi"("Euler Angles"=cluster{"phi":dbl, "theta":dbl, "psi":dbl} {"phi"=0.0, "theta"=90.0, "psi"=0.0}, "model in"=w36) -> ("model out"=w30:T2)  [unwired: 9 in]
      n22 = Unbundle By Name(w30) -> ("VertexList"=w33:T3[])
      n23 = Add(x=w33, y=T3 {"x"=-1.5, "y"=0.0, "z"=-4.0} ("point3f")) -> (x+y=w31:T3[])
      n24 = Bundle By Name(cluster=w30, "VertexList"=w31) -> (w29:T2)
    }
    frame "FreeCAD Sample" {
      w40 = T2 data[35798B] ("Model Out")
      n25 = Unbundle By Name(w40) -> ("VertexList"=w46:T3[])
      n26 = Divide(x=w46, y=40.0) -> (x/y=w44:cluster{"x":dbl, "y":dbl, "z":dbl}[])
      n27 = Bundle By Name(cluster=w40, "VertexList"=w44) -> (w43:T2)
      n28 = call "3DS Rotate Model.vi"("Euler Angles"=cluster{"phi":dbl, "theta":dbl, "psi":dbl} {"phi"=0.0, "theta"=180.0, "psi"=0.0}, "model in"=w43) -> ("model out"=w42:T2)  [unwired: 9 in]
    }
    frame "Schenkel" {
      w52 = T2 data[173558B] ("Model Out")
      n29 = Unbundle By Name(w52) -> ("VertexList"=w57:T3[])
      n30 = Divide(x=w57, y=44.0) -> (x/y=w55:cluster{"x":dbl, "y":dbl, "z":dbl}[])
      n31 = Bundle By Name(cluster=w52, "VertexList"=w55) -> (w54:T2)
      n32 = call "3DS Rotate Model.vi"("Euler Angles"=cluster{"phi":dbl, "theta":dbl, "psi":dbl} {"phi"=0.0, "theta"=90.0, "psi"=0.0}, "model in"=w54) -> ("model out"=w48:T2)  [unwired: 9 in]
      n33 = Unbundle By Name(w48) -> ("VertexList"=w51:T3[])
      n34 = Add(x=w51, y=T3 {"x"=0.0, "y"=0.0, "z"=-2.0} ("point3f")) -> (x+y=w49:T3[])
      n35 = Bundle By Name(cluster=w48, "VertexList"=w49) -> (w47:T2)
    }
    frame "Bunny" {
      w58 = T2 data[167846B] ("Model Out")
      n36 = Unbundle By Name(w58) -> ("VertexList"=w68:T3[])
      n37 = Divide(x=w68, y=44.0) -> (x/y=w66:cluster{"x":dbl, "y":dbl, "z":dbl}[])
      n38 = Bundle By Name(cluster=w58, "VertexList"=w66) -> (w65:T2)
      n39 = call "3DS Rotate Model.vi"("Euler Angles"=cluster{"phi":dbl, "theta":dbl, "psi":dbl} {"phi"=270.0, "theta"=180.0, "psi"=0.0}, "model in"=w65) -> ("model out"=w60:T2)  [unwired: 9 in]
      n40 = Unbundle By Name(w60) -> ("VertexList"=w63:T3[])
      n41 = Add(x=w63, y=T3 {"x"=0.0, "y"=0.0, "z"=-2.0} ("point3f")) -> (x+y=w61:T3[])
      n42 = Bundle By Name(cluster=w60, "VertexList"=w61) -> (w59:T2)
    }
    frame "Utah Teapot (Low Res)" {
      w69 = T2 data[172214B]  # Utah Teapot LR
      n43 = Unbundle By Name(w69) -> ("VertexList"=w79:T3[])
      n44 = Divide(x=w79, y=3.5) -> (x/y=w77:cluster{"x":dbl, "y":dbl, "z":dbl}[])
      n45 = Bundle By Name(cluster=w69, "VertexList"=w77) -> (w76:T2)
      n46 = call "3DS Rotate Model.vi"("Euler Angles"=cluster{"phi":dbl, "theta":dbl, "psi":dbl} {"phi"=270.0, "theta"=180.0, "psi"=0.0}, "model in"=w76) -> ("model out"=w71:T2)  [unwired: 9 in]
      n47 = Unbundle By Name(w71) -> ("VertexList"=w74:T3[])
      n48 = Add(x=w74, y=T3 {"x"=0.0, "y"=0.0, "z"=-1.5} ("point3f")) -> (x+y=w72:T3[])
      n49 = Bundle By Name(cluster=w71, "VertexList"=w72) -> (w70:T2)
    }
    frame "ASTM E2597 Step Wedge" {
      w80 = T2 data[14126B] ("Object Out")
      n50 = Unbundle By Name(w80) -> ("VertexList"=w90:T3[])
      n51 = Divide(x=w90, y=1.44) -> (x/y=w88:cluster{"x":dbl, "y":dbl, "z":dbl}[])
      n52 = Bundle By Name(cluster=w80, "VertexList"=w88) -> (w87:T2)
      n53 = call "3DS Rotate Model.vi"("Euler Angles"=cluster{"phi":dbl, "theta":dbl, "psi":dbl} {"phi"=90.0, "theta"=90.0, "psi"=180.0}, "model in"=w87) -> ("model out"=w82:T2)  [unwired: 9 in]
      n54 = Unbundle By Name(w82) -> ("VertexList"=w85:T3[])
      n55 = Add(x=w85, y=T3 {"x"=1.65, "y"=-1.0, "z"=0.0} ("point3f")) -> (x+y=w83:T3[])
      n56 = Bundle By Name(cluster=w82, "VertexList"=w83) -> (w81:T2)
    }
    frame "Corona Virus" {
      w92 = T2 {"VertexList"=array[27588 elements], "FaceList"=array[9196 elements], "NormalList"=array[27588 elements], "Mode"=enum."GL_TRIANGLES"} ("Object Out")
      n57 = Unbundle By Name(w92) -> ("VertexList"=w97:T3[])
      n58 = Divide(x=w97, y=3.0) -> (x/y=w91:cluster{"x":dbl, "y":dbl, "z":dbl}[])
      n59 = Add(x=w91, y=T3 {"x"=0.0, "y"=0.0, "z"=-2.0} ("point3f")) -> (x+y=w94:cluster{"x":dbl, "y":dbl, "z":dbl}[])
      n60 = Bundle By Name(cluster=w92, "VertexList"=w94) -> (w93:T2)
    }
    frame "Corona Virus (Low Res)" {
      w99 = T2 data[168014B] ("Object Out")
      n61 = Unbundle By Name(w99) -> ("VertexList"=w104:T3[])
      n62 = Divide(x=w104, y=3.0) -> (x/y=w100:cluster{"x":dbl, "y":dbl, "z":dbl}[])
      n63 = Add(x=w100, y=T3 {"x"=0.0, "y"=0.0, "z"=-2.0} ("point3f")) -> (x+y=w101:cluster{"x":dbl, "y":dbl, "z":dbl}[])
      n64 = Bundle By Name(cluster=w99, "VertexList"=w101) -> (w98:T2)
    }
    frame "Offset" {
      w105 = T2 data[54782B] ("Model Out")
      n65 = Unbundle By Name(w105) -> ("VertexList"=w111:T3[])
      n66 = Divide(x=w111, y=3.0) -> (x/y=w107:cluster{"x":dbl, "y":dbl, "z":dbl}[])
      n67 = Add(x=w107, y=T3 {"x"=0.0, "y"=0.0, "z"=-2.0} ("point3f")) -> (x+y=w108:cluster{"x":dbl, "y":dbl, "z":dbl}[])
      n68 = Bundle By Name(cluster=w105, "VertexList"=w108) -> (w106:T2)
    }
  }
  "Model Out" <- w2
